vi "InitWSMessageBroker.vi"(7 "Server Controller Enqueuer":refnum<class "Message Enqueuer.lvclass">, 8 "error in (no error)":errorcluster, 9 "Websocket Client Handler":refnum<class "WS Client.lvclass">, 10 "Listen Port":u16, 11 "Broker Name":string) -> (0 "error out":errorcluster, 2 "Broadcast Message Transport":refnum<class "Message Transport Queue.lvclass">, 3 "Websocket Message Broker Interface Ref out":refnum<class "WS Message Broker Interface Ref.lvclass">)   [LabVIEW 2016, in "WebSocket Networking.lvlib" / "WS Message Broker Interface Ref.lvclass"]
doc: "--\nCopyright © 2017 Composed SystemsI All rights reserved.\n\nAuthor: Jon McBee <jon.mcbee@composed.io>\n\nThis library is provided \"AS IS\" ,WITHOUT WARRANTIES OR\nCONDITIONS OF ANY KIND, either express or implied.\n\nComposed Systems -- composed.io\n\nStream 0.0.1.1\nJon McBee - Composed Systems\nCopyright (c) 2017, Composed Systems"
uses:
  <userlib>/Common Components/WebSocket Networking/WS Message Broker Interface Ref/WS Message Broker Interface Ref.lvclass
  C:/Program Files (x86)/National Instruments/LabVIEW 2016/user.lib/Composed Systems/Stream/Mediator/Classes/Message Broker Interface Ref/Message Broker Interface Ref.lvclass
  C:/Program Files (x86)/National Instruments/LabVIEW 2016/user.lib/Composed Systems/Stream/Mediator/Classes/Message Broker Interface/Message Broker Interface.lvclass
  C:/Program Files (x86)/National Instruments/LabVIEW 2016/user.lib/Composed Systems/Stream/Mediator/Classes/Websocket Message Broker Interface Ref/Websocket Message Broker Interface Ref.lvclass
  <userlib>/Common Components/WebSocket Networking/WS Client/WS Client.lvclass
  C:/Program Files (x86)/National Instruments/LabVIEW 2016/user.lib/Composed Systems/Stream/Mediator/Classes/Websocket Client Handler Actor/Websocket Client Handler/Websocket Client Handler.lvclass
  <vilib>/ActorFramework/Message Enqueuer/Message Enqueuer.lvclass
  <userlib>/Composed Systems/Stream/Mediator/Classes/Message Transport Queue/Message Transport Queue.lvclass
  <userlib>/Composed Systems/Stream/Mediator/Classes/Websocket Topic Actor/Websocket Topic Actor.lvclass
  <userlib>/Common Components/WebSocket Networking/WS Server/WS Server.lvclass
  C:/Program Files (x86)/National Instruments/LabVIEW 2016/user.lib/Composed Systems/Stream/Mediator/Classes/Websocket Server Actor/Websocket Server/Websocket Server.lvclass
  C:/Program Files (x86)/National Instruments/LabVIEW 2016/user.lib/Composed Systems/Stream/Mediator/Classes/Mediated Asynchronous Actor/Mediated Asynchronous Actor.lvclass
  <userlib>/Composed Systems/Stream/Mediator/Classes/Websocket Server Actor/Websocket Server/Websocket Server.lvclass/Websocket Server.ctl
  <userlib>/Common Components/WebSocket Networking/WS Server/WS Server.lvclass/WS Server.ctl
  <userlib>/Composed Systems/Stream/Mediator/Classes/Websocket Message Broker Interface Ref/Websocket Message Broker Interface Ref.lvclass/Websocket Message Broker Interface Ref.ctl
  <userlib>/Composed Systems/Stream/Mediator/Classes/Websocket Message Broker/Websocket Message Broker.lvclass
  C:/Program Files (x86)/National Instruments/LabVIEW 2016/user.lib/Composed Systems/Stream/Mediator/Classes/Message Broker/Message Broker.lvclass
  <userlib>/Composed Systems/Stream/Mediator/Classes/Message Broker Interface Ref/Message Broker Interface Ref.lvclass
  <userlib>/Composed Systems/Stream/Mediator/Classes/Websocket Server Actor/Websocket Server/Websocket Server.lvclass
  <userlib>/Composed Systems/Stream/Mediator/Classes/Mediated Asynchronous Actor/Mediated Asynchronous Actor.lvclass
  <userlib>/Composed Systems/Stream/Mediator/Classes/Websocket Message Broker Interface Ref/Websocket Message Broker Interface Ref.lvclass
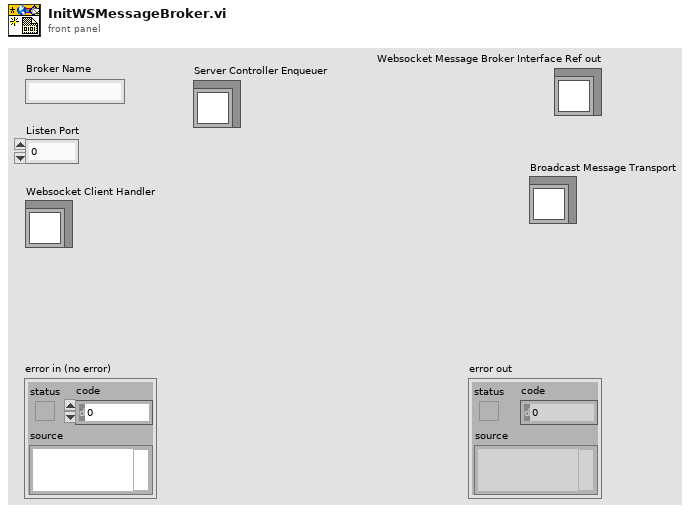
[diagram p1: front panel]
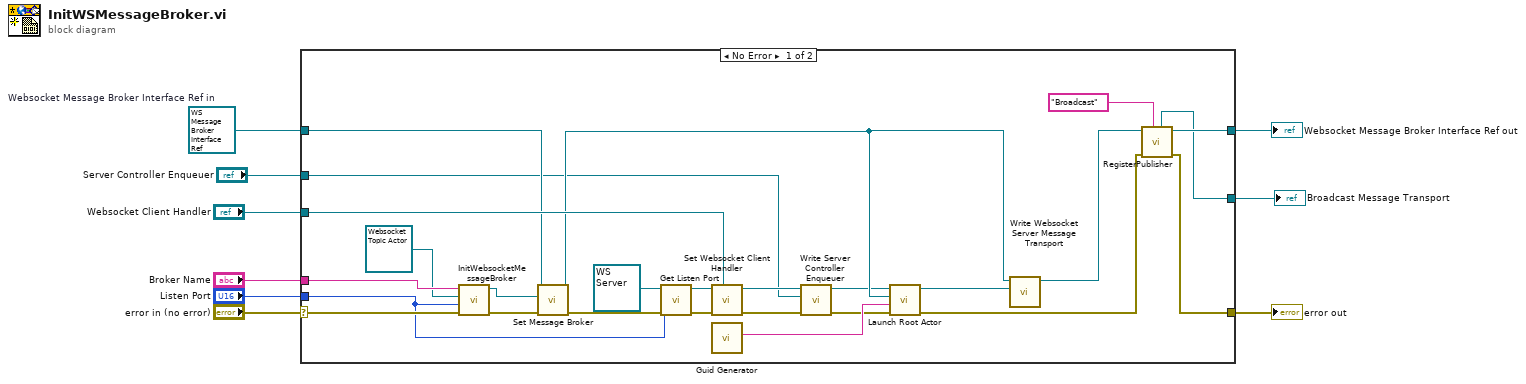
[diagram p0: block diagram]
diagram:
  w7 = refnum<class "WS Message Broker Interface Ref.lvclass"> refnum  # Websocket Message Broker Interface Ref in
  n1 = case shown="No Error" "error in (no error)" {
    selector: "error in (no error)" -> [w35 w37]
    tunnel: [w11 w37] -> w8
    tunnel: [w14 w36] -> w3
    tunnel: w7 -> [w28 w36]
    tunnel: "Broker Name" -> [w34 _]
    tunnel: "Listen Port" -> [w23 _]
    tunnel: "Websocket Client Handler" -> [w30 _]
    tunnel: "Server Controller Enqueuer" -> [w15 _]
    tunnel: [w10 _] -> w1
    frame No Error {
      n2 = call <userlib>:"InitWebsocketMessageBroker.vi"("error in (no error)"=w35, "Listen Port"=w23, "Websocket Topic Actor"=refnum<class "Websocket Topic Actor.lvclass"> refnum, "Broker Name"=w34) -> ("error out"=w32:errorcluster, "Message Broker Ref"=w31:refnum<data-value>)  [unwired: 6 in]
      n3 = call <userlib>:"Set Message Broker.vi"("error in (no error)"=w32, "Broker"=w31, "Message Broker Interface Ref in"=w28) -> ("error out"=w27:errorcluster, "Message Broker Interface Ref out"=w20:refnum<class "WS Message Broker Interface Ref.lvclass">)  [unwired: 7 in]
      n4 = call <userlib>:"Get Listen Port.vi"("error in (no error)"=w27, "Listen Port"=w23, "Websocket Server in"=refnum<class "WS Server.lvclass"> refnum ("Websocket Server.lvclass")) -> ("error out"=w26:errorcluster, "Websocket Server out"=w24:refnum<class "WS Server.lvclass">)  [unwired: 7 in]
      n5 = call <userlib>:"Set Websocket Client Handler.vi"("Websocket Client Handler"=w30, "error in (no error)"=w26, "Websocket Server in"=w24) -> ("error out"=w29:errorcluster, "Websocket Server out"=w17:refnum<class "WS Server.lvclass">)  [unwired: 7 in]
      n6 = call <vilib>:"Guid Generator.vi"() -> ("GUID"=w22:string)  [unwired: 10 in, 1 out]
      n7 = call <userlib>:"Write Server Controller Enqueuer.vi"("error in (no error)"=w29, "Actor Framework:Message Enqueuer"=w15, "WS Server in"=w17) -> ("error out"=w18:errorcluster, "WS Server out"=w16:refnum<class "WS Server.lvclass">)  [unwired: 7 in]
      n8 = call <userlib>:"Launch Root Actor.vi"("error in (no error)"=w18, "Actor Name"=w22, "Message Broker"=w20, "Mediated Asynchronous Actor in"=w16) -> ("error out"=w12:errorcluster, "Command Actor Message Transport"=w21:refnum<class "Message Transport Interface.lvclass">)  [unwired: 6 in]
      n9 = call <userlib>:"Write Websocket Server Message Transport.vi"("Stream Mediator.lvlib:Message Transport Interface.lvclass"=w21, "Websocket Message Broker Interface Ref in"=w20) -> ("Websocket Message Broker Interface Ref out"=w19:refnum<class "WS Message Broker Interface Ref.lvclass">)  [unwired: 9 in]
      n10 = call-dynamic "RegisterPublisher.vi"("Topic Name"="Broadcast", "error in (no error)"=w12, "Message Broker Interface Ref in"=w19) -> ("error out"=w11:errorcluster, "Message Broker Interface Ref out"=w14:refnum<class "WS Message Broker Interface Ref.lvclass">, "Transport"=w10:refnum<class "Message Transport Queue.lvclass">)  [unwired: 4 in, 2 out]
    }
    frame Error {
    }
  }
  "error out" <- w8
  "Websocket Message Broker Interface Ref out" <- w3
  "Broadcast Message Transport" <- w1
